vi "Run_Python_Command.vi"(8 "error in":errorcluster, 11 "Functions":T1=enum."HMS_IPConfig_Conflict_IP") -> (0 "error out":errorcluster, 2 "Standard Output":string, 3 "Output":bool)   [LabVIEW 2025]
uses:
  Control/Python Function.ctl
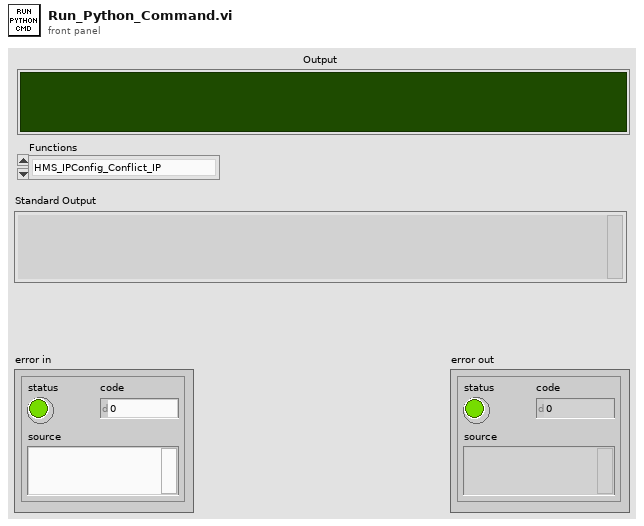
[diagram p1: front panel]
types:
  T1 = typedef "Python Function.ctl" = enum16{"HMS_IPConfig", "HMS_IPConfig_Verify_DHCP_Enabled", "HMS_IPConfig_Conflict_IP"}
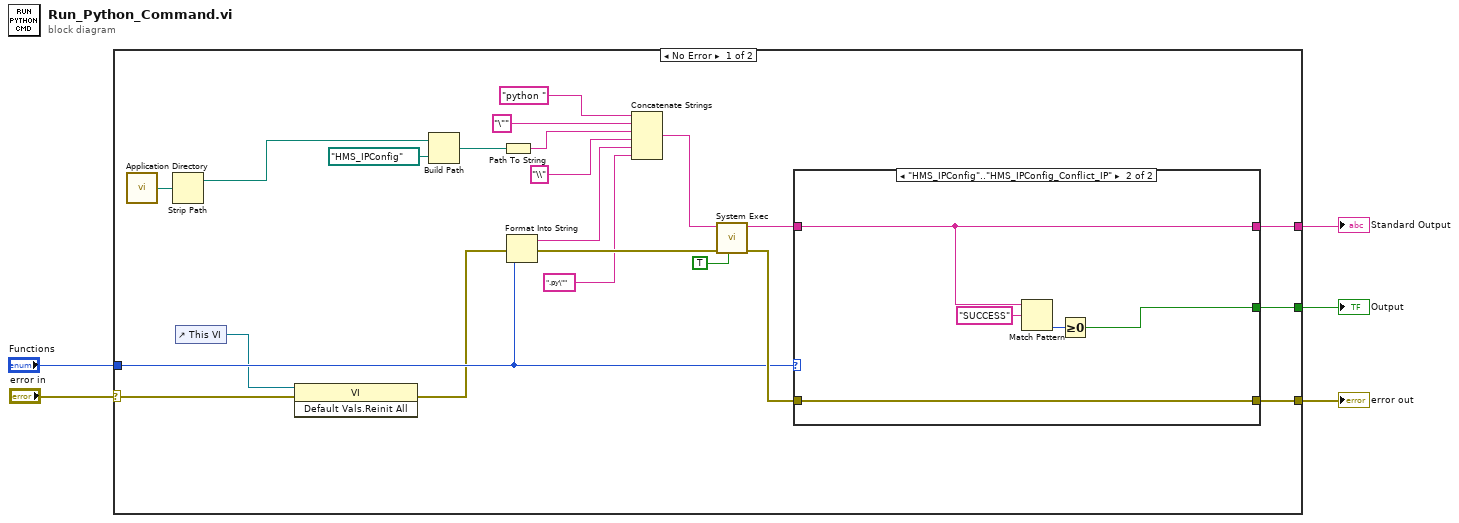
[diagram p0: block diagram]
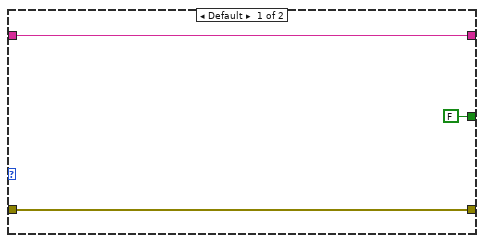
[diagram p2: hidden frame]
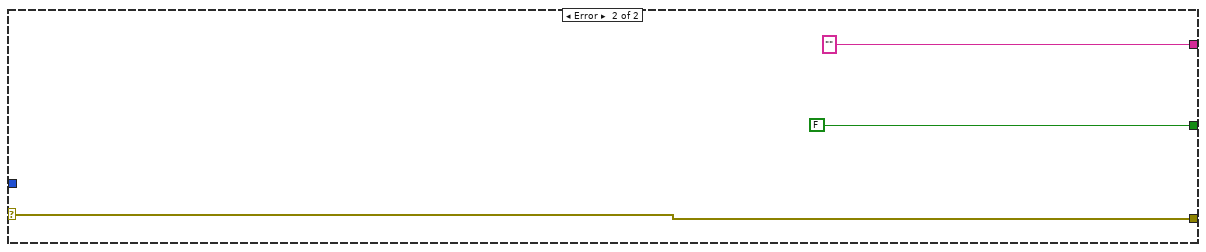
[diagram p3: hidden frame]
diagram:
  n1 = case shown="No Error" "error in" {
    selector: "error in" -> [w7 w38]
    tunnel: [w21 w38] -> w4
    tunnel: "Functions" -> [w20 _]
    tunnel: [w18 "" ("standard output")] -> w3
    tunnel: [w19 FALSE] -> w2
    frame No Error {
      n2 = call <vilib>:"Application Directory.vi"() -> ("Application Directory"=w27:path)
      n3 = Strip Path(path=w27) -> (stripped path=w16:path)  [unwired: 1 out]
      n4 = control-ref of="This VI"() -> (w8:refnum<vi>)
      n5 = invoke class="VI" method="Default Vals.Reinit All"(reference=w8, error in=w7) -> (error out=w6:errorcluster)  [unwired: 1 in, 2 out]
      n6 = Build Path(base path=w16, name or relative path=path "HMS_IPConfig") -> (appended path=w25:path)
      n7 = Path To String(path=w25) -> (string=w26:string)
      n8 = Format Into String(error in=w6, w20) -> (resulting string=w13:string, error out=w23:errorcluster)  [unwired: 2 in]
      n9 = Concatenate Strings("python " ("string"), "\"" ("string"), w26, "\\" ("string"), w13, ".py\"" ("string")) -> (w9:string)
      n10 = call <vilib>:"System Exec.vi"("run minimized? (F)"=TRUE, "error in (no error)"=w23, "command line"=w9) -> ("error out"=w22:errorcluster, "standard output"=w17:string)  [unwired: 5 in, 2 out]
      n11 = case shown="\"HMS_IPConfig\"..\"HMS_IPConfig_Conflict_IP\"" w20 {
        tunnel: [FALSE w32] -> w19
        tunnel: w22 -> [w30 w33]
        tunnel: [w30 w33] -> w21
        tunnel: [w29 w31] -> w18
        tunnel: w17 -> [w29 w31]
        frame Default {
        }
        frame "HMS_IPConfig".."HMS_IPConfig_Conflict_IP" {
          n12 = Match Pattern(string=w31, regular expression="SUCCESS") -> (offset past match=w34:i32)  [unwired: 1 in, 3 out]
          n13 = Greater Or Equal To 0?(x=w34) -> (x >= 0?=w32:bool)
        }
      }
    }
    frame Error {
    }
  }
  "error out" <- w4
  "Standard Output" <- w3
  "Output" <- w2
